vi "setUp.vi"(8 "error in (no error)":errorcluster, 11 "reference in":refnum<class "Scripting.lvclass">) -> (0 "error out":errorcluster, 3 "reference out":refnum<class "Scripting.lvclass">)   [LabVIEW 2020, in "Scripting.lvclass"]
doc: "setUp runs prior to the test method during test execution. Use this method to initialize any object data required by your tests."
uses:
  Scripting.lvclass
  C:/dev/git/niveristand-custom-device-testing-tools/VeriStandScriptingTestCase/VeriStandScriptingTestCase.lvclass
  C:/Program Files (x86)/National Instruments/LabVIEW 2020/vi.lib/addons/_JKI Toolkits/VI Tester/TestCase.llb/TestCase.lvclass
  <vilib>/addons/_JKI Toolkits/VI Tester/TestCase.llb/TestCase.lvclass
  niveristand-custom-device-testing-tools/VeriStandScriptingTestCase/VeriStandScriptingTestCase.lvclass
  C:/dev/git/niveristand-aim-milStd1553-custom-device/Source/Custom Device Support/Tests/Unit/Scripting/Scripting.lvclass
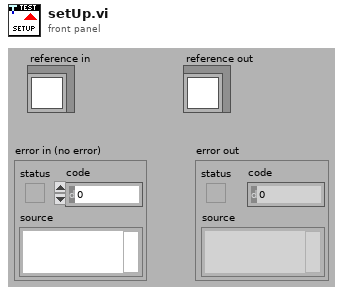
[diagram p1: front panel]
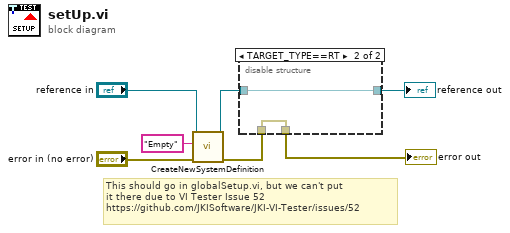
[diagram p0: block diagram]
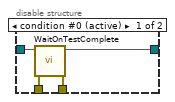
[diagram p2: hidden frame]
diagram:
  # "This should go in globalSetup.vi, but we can't put\nit there due to VI Tester Issue 52\nhttps://github.com/JKISoftware/JKI-VI-Tester/issues/52"
  n1 = call "CreateNewSystemDefinition.vi"("error in (no error)"="error in (no error)", "System Definition Name"="Empty", "VeriStandScriptingTestCase in"="reference in") -> ("error out"=w4:errorcluster, "VeriStandScriptingTestCase out"=w2:refnum<class "Scripting.lvclass">)  [unwired: 7 in]
  n2 = disable-structure shown="TARGET_TYPE==RT" {
    disable-tunnel: w4 -> [w11 w12]
    disable-tunnel: [w10 w12] -> w7
    disable-tunnel: [w9 w13] -> w6
    disable-tunnel: w2 -> [w8 w13]
    frame condition #0 (active) {
      n3 = call <vilib>:"WaitOnTestComplete.vi"("error in (no error)"=w11, "TestCase in"=w8) -> ("error out"=w10:errorcluster, "TestCase out"=w9:refnum<class "Scripting.lvclass">)  [unwired: 8 in]
    }
    frame condition #1 {
    }
  }
  "error out" <- w7
  "reference out" <- w6
